vi "Configure Mathematics.vi"(0 "VISA resource name":refnum<visa-resource-name>, 1 "K (1)":dbl=1.0, 2 "L (0)":dbl, 3 "M (1)":dbl=1.0, 5 "Mathematics State (T: On)":bool=TRUE, 7 "Mathematical Expression (0: ((K * X) + L))":i32(ring) items=["((K * X) + L)", "((K / X) + L)", "(((K * X) + L) / M)", "(((K / X) + L) / M)"], 11 "error in (no error)":errorcluster) -> (4 "VISA resource name out":refnum<visa-resource-name>, 15 "error out":errorcluster)   [LabVIEW 2019, in "Pendulum CNT90.lvlib"]
doc: "Switches on/off the mathematical function and defines the mathematical expression used for mathematical operations."
uses:
  Pendulum CNT90.lvlib
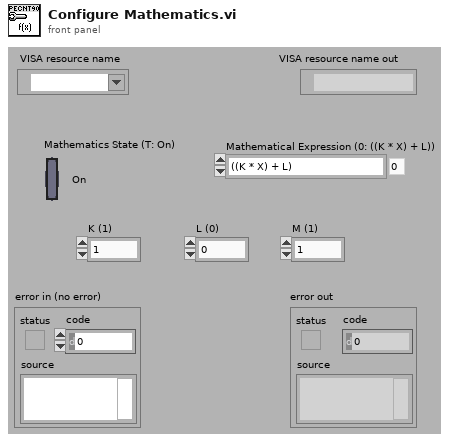
[diagram p1: front panel]
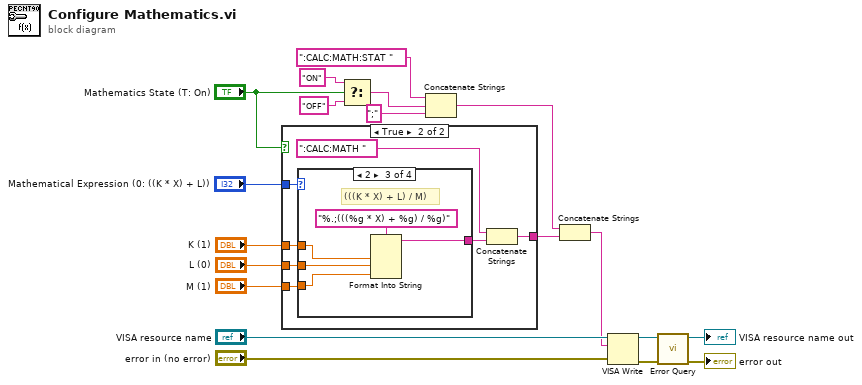
[diagram p0: block diagram]
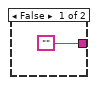
[diagram p2: hidden frame]
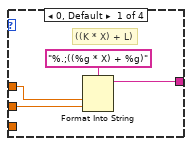
[diagram p3: hidden frame]
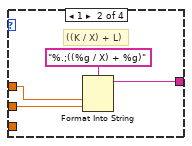
[diagram p4: hidden frame]
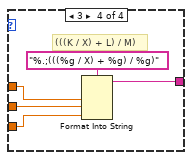
[diagram p5: hidden frame]
diagram:
  n1 = case shown="True" "Mathematics State (T: On)" {
    tunnel: "Mathematical Expression (0: ((K * X) + L))" -> [_ w27]
    tunnel: "K (1)" -> [_ w26]
    tunnel: "L (0)" -> [_ w25]
    tunnel: "M (1)" -> [_ w24]
    tunnel: ["" w21] -> w2
    frame False {
    }
    frame True {
      n2 = case shown="2" w27 {
        tunnel: w26 -> [w30 w33 w38 w43]
        tunnel: w25 -> [w29 w32 w37 w42]
        tunnel: [w28 w34 w39 w44] -> w22
        tunnel: w24 -> [_ _ w36 w41]
        frame 0, Default {
          # "((K * X) + L)"
          n3 = Format Into String(format string="%.;((%g * X) + %g)", w30, w29) -> (resulting string=w28:string)  [unwired: 2 in, 1 out]
        }
        frame 1 {
          # "((K / X) + L)"
          n4 = Format Into String(format string="%.;((%g / X) + %g)", w33, w32) -> (resulting string=w34:string)  [unwired: 2 in, 1 out]
        }
        frame 2 {
          # "(((K * X) + L) / M)"
          n5 = Format Into String(format string="%.;(((%g * X) + %g) / %g)", w38, w37, w36) -> (resulting string=w39:string)  [unwired: 2 in, 1 out]
        }
        frame 3 {
          # "(((K / X) + L) / M)"
          n6 = Format Into String(format string="%.;(((%g / X) + %g) / %g)", w43, w42, w41) -> (resulting string=w44:string)  [unwired: 2 in, 1 out]
        }
      }
      n7 = Concatenate Strings(":CALC:MATH ", w22) -> (w21:string)
    }
  }
  n8 = Select(t="ON", s="Mathematics State (T: On)", f="OFF") -> (s? t:f=w10:string)
  n9 = Concatenate Strings(":CALC:MATH:STAT ", w10, ";" ("string")) -> (w3:string)
  n10 = Concatenate Strings(w3, w2) -> (w4:string)
  n11 = VISA Write(VISA resource name="VISA resource name", write buffer=w4, error in (no error)="error in (no error)") -> (VISA resource name out=w17:refnum<visa-resource-name>, error out=w14:errorcluster)  [unwired: 1 out]
  n12 = call "Error Query.vi"("error in (no error)"=w14, "VISA resource name"=w17) -> ("error out"=→"error out":errorcluster, "VISA resource name out"=→"VISA resource name out":refnum<visa-resource-name>)  [unwired: 6 in, 2 out]
